vi "Receive_Log_File_FGV.vi"(7 "Session name":string, 8 "error in (no error)":errorcluster, 9 "Command":enum16{"Initialize", "Update", "Stop"}(ring), 10 "Time (ms)":u32, 11 "Processed bytes":u8[](array[numeric])) -> (0 "error out":errorcluster, 3 "Receive Log File Path":path)   [LabVIEW 2017]
uses:
  <vilib>/Utility/file.llb/Write Delimited Spreadsheet (string).vi
  <vilib>/Utility/file.llb/Write Delimited Spreadsheet (I64).vi
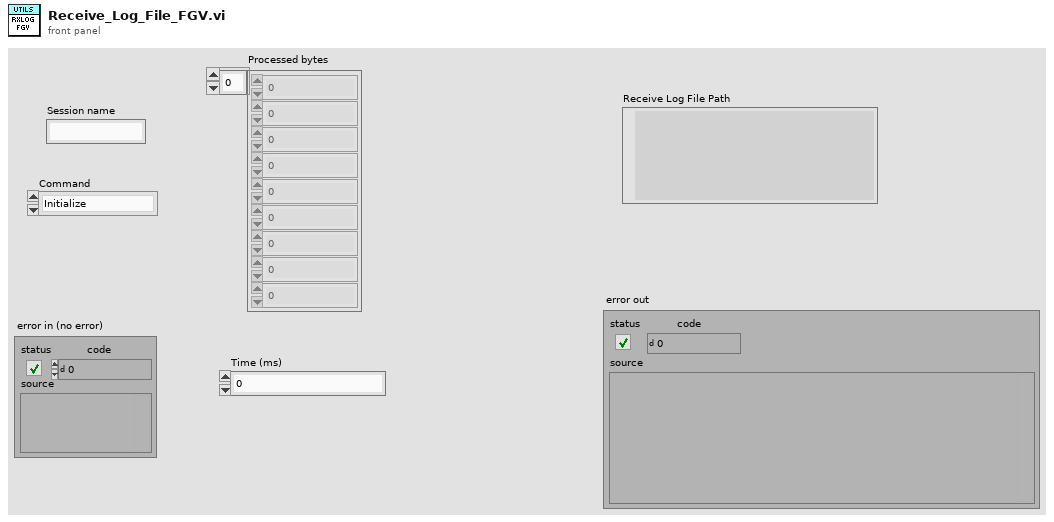
[diagram p1: front panel]
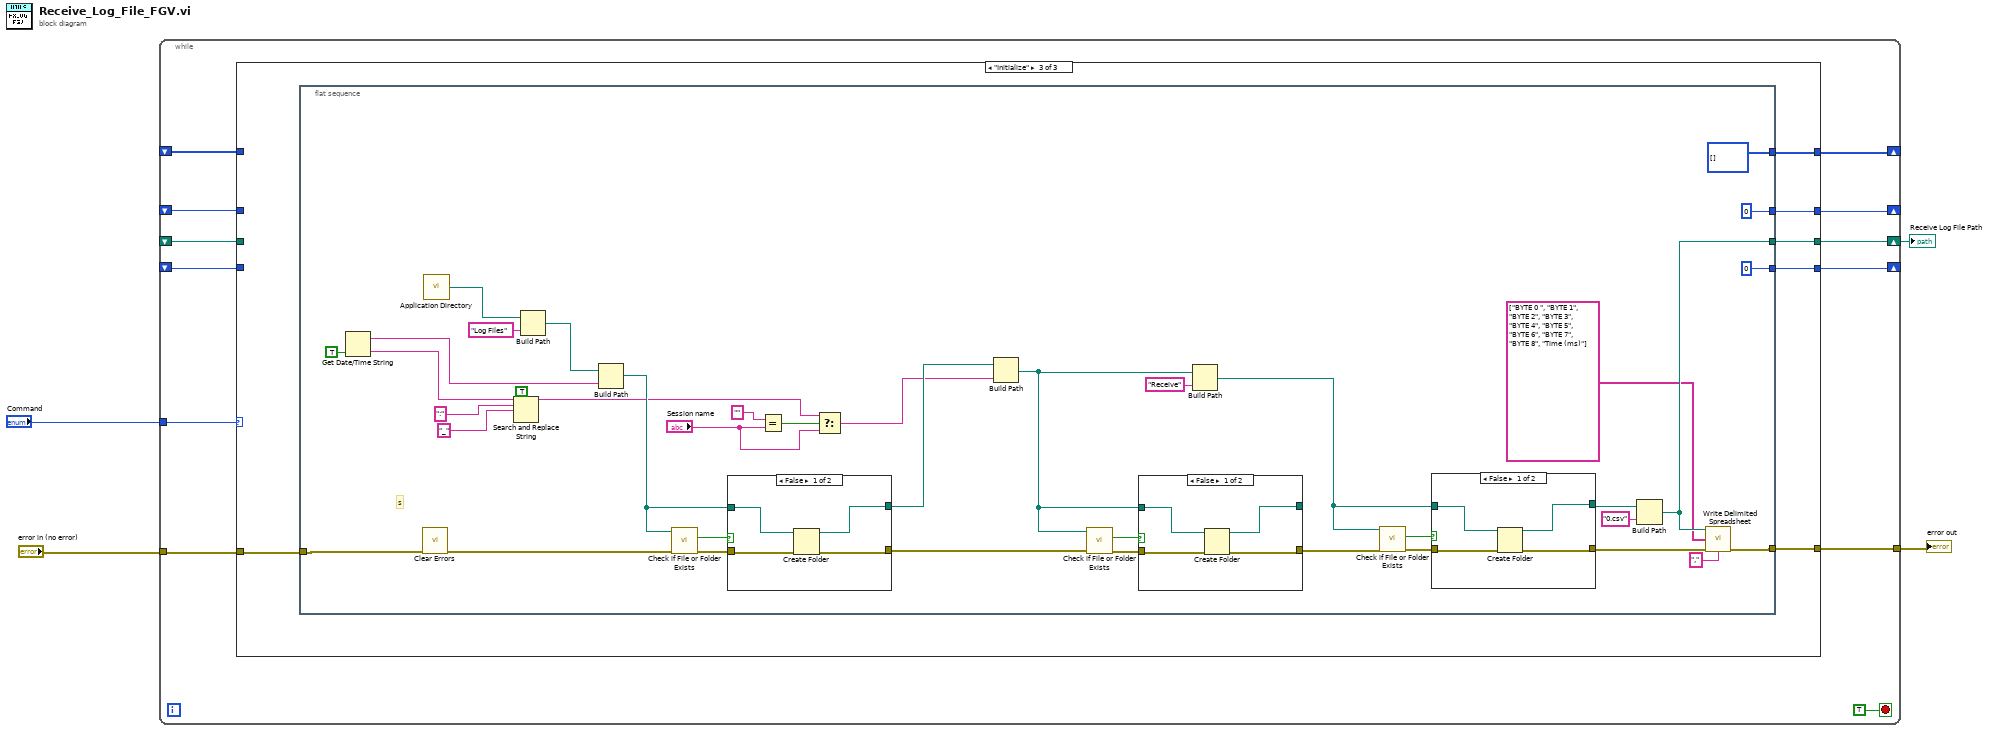
[diagram p0: block diagram]
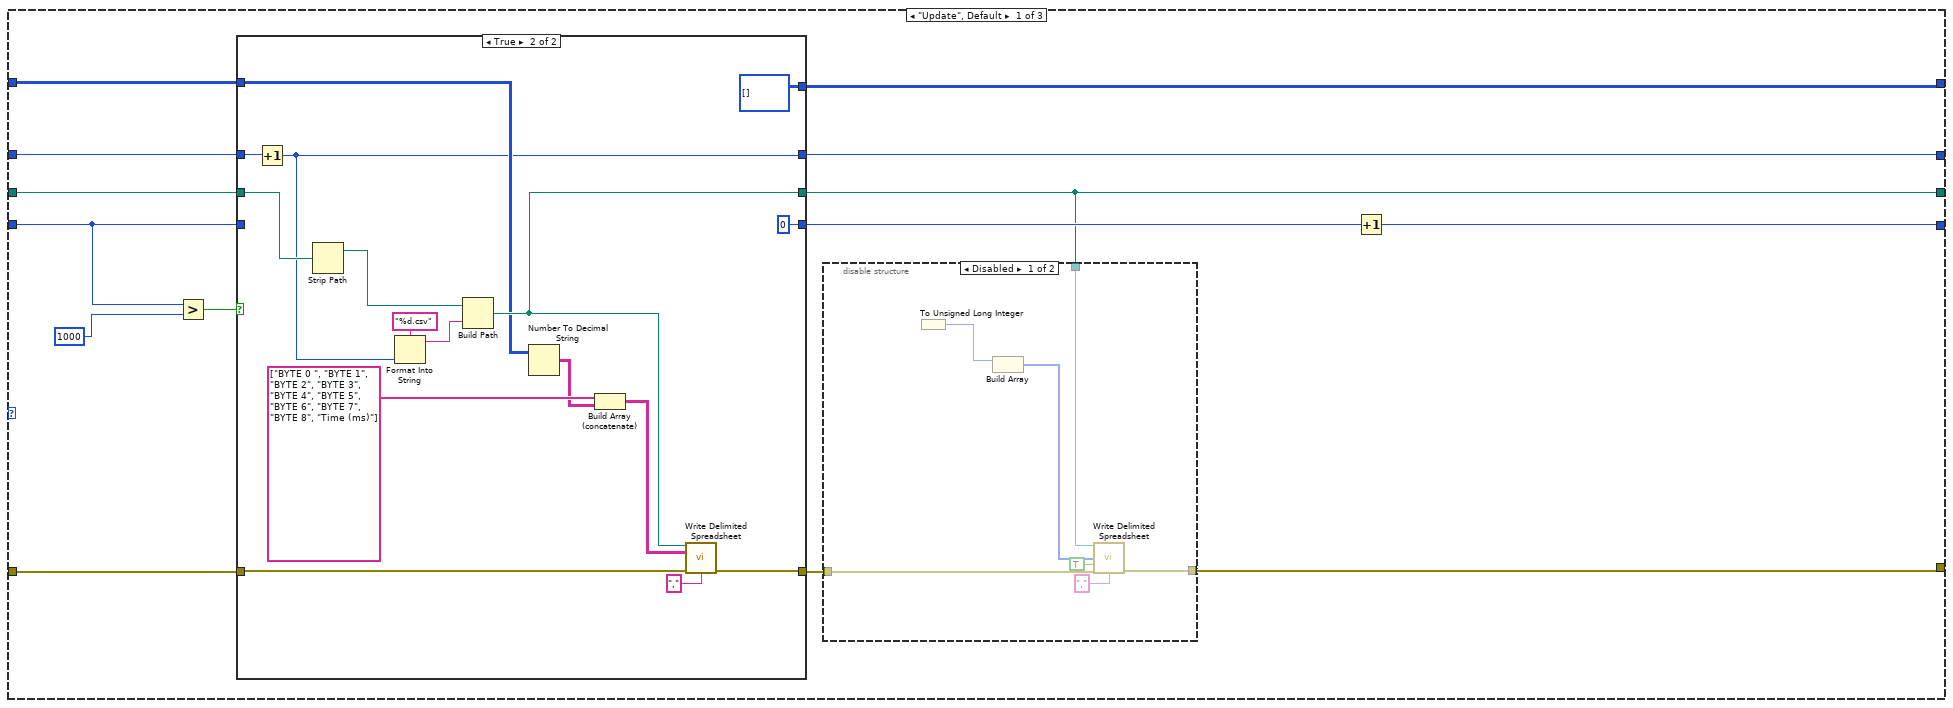
[diagram p2: hidden frame]
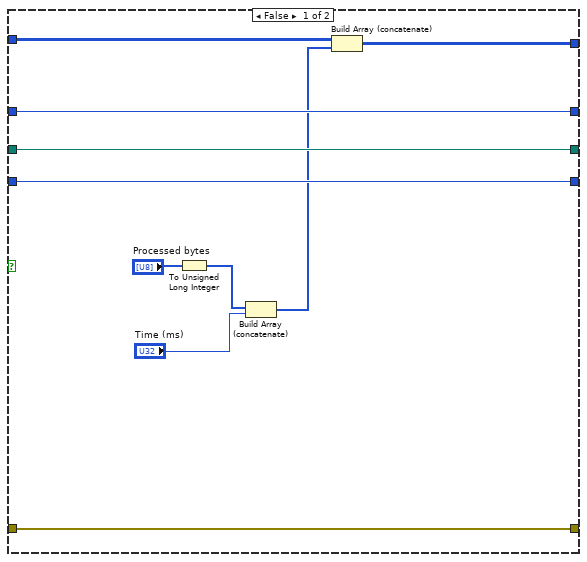
[diagram p4: hidden frame]
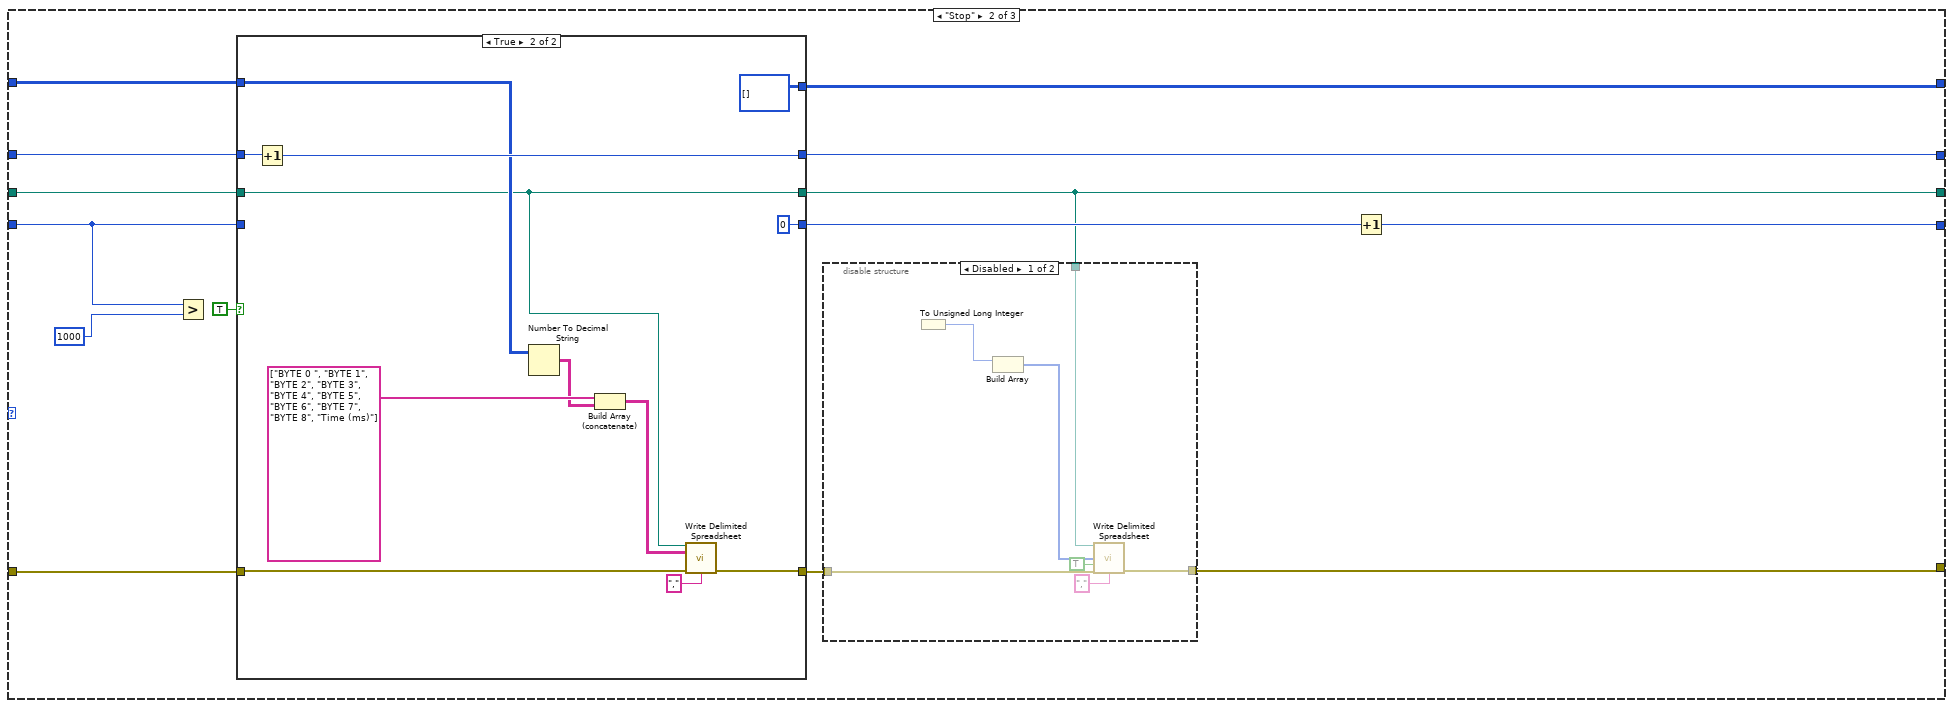
[diagram p5: hidden frame]
diagram:
  n1 = while {
    tunnel: "error in (no error)" -> [w16]
    tunnel: "Command" -> [w15]
    tunnel: [w13] -> w2
    shift-right: [w12] -> w3
    shift-left: _ -> [w9]
    shift-right: [w11] -> _
    shift-left: _ -> [w10]
    shift-right: [w8] -> _
    shift-left: _ -> [w7]
    shift-right: [w6] -> _
    shift-left: _ -> [w5]
    stop <- TRUE stop-if-true
    n2 = case shown="\"Initialize\"" w15 {
      tunnel: w16 -> [w30 w80 w113]
      tunnel: [w20 w71 w112] -> w13
      tunnel: [w21 w72 w111] -> w12
      tunnel: [w19 w70 w110] -> w11
      tunnel: w10 -> [w24 w75 _]
      tunnel: w9 -> [w27 w78 _]
      tunnel: [w25 w76 w109] -> w8
      tunnel: w7 -> [w26 w77 _]
      tunnel: [w17 w68 w108] -> w6
      tunnel: w5 -> [w18 w69 _]
      frame "Update", Default {
        n3 = Greater?(x=w24, y=1000) -> (0:w29:bool)
        n4 = case shown="True" w29 {
          tunnel: w30 -> [w49 w62]
          tunnel: [w49 w60] -> w22
          tunnel: w27 -> [w50 w66]
          tunnel: [w50 w59] -> w21
          tunnel: w26 -> [w48 w56]
          tunnel: [w48 w51] -> w25
          tunnel: w24 -> [w47 _]
          tunnel: [w47 0] -> w23
          tunnel: w18 -> [w43 w55]
          tunnel: [w41 u32[][] []] -> w17
          frame False {
            n5 = To Unsigned Long Integer(number="Processed bytes") -> (unsigned 32bit integer=w45:u32[])
            n6 = Build Array (concatenate)(w45, "Time (ms)") -> (w42:u32[])
            n7 = Build Array (concatenate)(w43, w42) -> (w41:u32[][])
          }
          frame True {
            n8 = Increment(x=w56) -> (x+1=w51:i32)
            n9 = Strip Path(path=w66) -> (stripped path=w65:path)  [unwired: 1 out]
            n10 = Format Into String(format string="%d.csv", w51) -> (resulting string=w63:string)  [unwired: 2 in, 1 out]
            n11 = Build Path(base path=w65, name or relative path=w63) -> (appended path=w59:path)
            n12 = Number To Decimal String(number=w55) -> (decimal integer string=w53:string[][])  [unwired: 1 in]
            n13 = Build Array (concatenate)(string[] ["BYTE 0 ", "BYTE 1", "BYTE 2", "BYTE 3", "BYTE 4", "BYTE 5", "BYTE 6", "BYTE 7", "BYTE 8", "Time (ms)"], w53) -> (w52:string[][])
            n14 = call-poly <vilib>:"Write Delimited Spreadsheet.vi"("file path (dialog if empty)"=w59, "2D data"=w52, "error in (no error)"=w62, "delimiter (\\t)"="," ("delimiter (\\t)")) -> ("error out"=w60:errorcluster)  [unwired: 10 in, 1 out]
          }
        }
        n15 = disable-structure shown="Disabled" {
          disable-tunnel: w22 -> [w39 w40]
          disable-tunnel: w21 -> [w38 _]
          disable-tunnel: [w35 w40] -> w20
          frame Disabled {
            n16 = To Unsigned Long Integer() -> (number=w34:u32, unsigned 32bit integer=w33:u32)
            n17 = Build Array(w33) -> (w31:u32[], w32:u32)
            n18 = call-poly <vilib>:"Write Delimited Spreadsheet.vi"("file path (dialog if empty)"=w38, "1D data"=w31, "append to file? (new file:F)"=TRUE, "error in (no error)"=w39, "delimiter (\\t)"="," ("delimiter (\\t)")) -> ("error out"=w35:errorcluster)  [unwired: 9 in, 1 out]
          }
          frame Enabled {
          }
        }
        n19 = Increment(x=w23) -> (x+1=w19:i32)
      }
      frame "Stop" {
        n20 = Greater?(x=w75, y=1000) -> ()  [unwired: 1 out]
        n21 = case shown="True" TRUE {
          tunnel: w80 -> [w94 w106]
          tunnel: [w94 w104] -> w73
          tunnel: w78 -> [w95 w96]
          tunnel: [w95 w96] -> w72
          tunnel: w77 -> [w93 w101]
          tunnel: [w93 w107] -> w76
          tunnel: w75 -> [w92 _]
          tunnel: [w92 0] -> w74
          tunnel: w69 -> [w91 w100]
          tunnel: [w91 u32[][] []] -> w68
          frame False {
          }
          frame True {
            n22 = Increment(x=w101) -> (x+1=w107:i32)
            n23 = Number To Decimal String(number=w100) -> (decimal integer string=w98:string[][])  [unwired: 1 in]
            n24 = Build Array (concatenate)(string[] ["BYTE 0 ", "BYTE 1", "BYTE 2", "BYTE 3", "BYTE 4", "BYTE 5", "BYTE 6", "BYTE 7", "BYTE 8", "Time (ms)"], w98) -> (w97:string[][])
            n25 = call-poly <vilib>:"Write Delimited Spreadsheet.vi"("file path (dialog if empty)"=w96, "2D data"=w97, "error in (no error)"=w106, "delimiter (\\t)"="," ("delimiter (\\t)")) -> ("error out"=w104:errorcluster)  [unwired: 10 in, 1 out]
          }
        }
        n26 = disable-structure shown="Disabled" {
          disable-tunnel: w73 -> [w89 w90]
          disable-tunnel: w72 -> [w88 _]
          disable-tunnel: [w85 w90] -> w71
          frame Disabled {
            n27 = To Unsigned Long Integer() -> (number=w84:u32, unsigned 32bit integer=w83:u32)
            n28 = Build Array(w83) -> (w81:u32[], w82:u32)
            n29 = call-poly <vilib>:"Write Delimited Spreadsheet.vi"("file path (dialog if empty)"=w88, "1D data"=w81, "append to file? (new file:F)"=TRUE, "error in (no error)"=w89, "delimiter (\\t)"="," ("delimiter (\\t)")) -> ("error out"=w85:errorcluster)  [unwired: 9 in, 1 out]
          }
          frame Enabled {
          }
        }
        n30 = Increment(x=w74) -> (x+1=w70:i32)
      }
      frame "Initialize" {
        n31 = flat-sequence {
          tunnel: w113 -> [w115]
          tunnel: [w125] -> w112
          tunnel: [w127] -> w111
          tunnel: [0] -> w110
          tunnel: [0] -> w109
          tunnel: [u32[][] []] -> w108
          frame #0 {
            # "s"
            n32 = Get Date/Time String(want seconds? (F)=TRUE) -> (date string=w148:string, time string=w143:string)  [unwired: 2 in]
            n33 = call <vilib>:"Clear Errors.vi"("error in (no error)"=w115) -> ("error out"=w114:errorcluster)  [unwired: 5 in, 1 out]
            n34 = call <vilib>:"Application Directory.vi"() -> ("Application Directory"=w151:path)
            n35 = Search and Replace String(replace all?=TRUE ("replace all? (F)"), input string=w143, search string=":", replace string="_" ("replace string (\"\")")) -> (result string=w119:string)  [unwired: 4 in, 3 out]
            n36 = Build Path(base path=w151, name or relative path="Log Files") -> (appended path=w149:path)
            n37 = Build Path(base path=w149, name or relative path=w148) -> (appended path=w145:path)
            n38 = call <vilib>:"Check if File or Folder Exists.vi"("error in (no error)"=w114, "path"=w145) -> ("error out"=w146:errorcluster, "file or folder exists?"=w147:bool)  [unwired: 7 in, 1 out]
            n39 = case shown="False" w147 {
              tunnel: w146 -> [w168 w170]
              tunnel: [w166 w170] -> w137
              tunnel: w145 -> [w167 w169]
              tunnel: [w165 w169] -> w144
              frame False {
                n40 = Create Folder(path (use dialog)=w167, error in=w168) -> (created path=w165:path, error out=w166:errorcluster)  [unwired: 1 in, 1 out]
              }
              frame True {
              }
            }
            n41 = Equal?(x="", y="Session name") -> (x = y?=w120:bool)
            n42 = Select(t=w119, s=w120, f="Session name") -> (s? t:f=w118:string)
            n43 = Build Path(base path=w144, name or relative path=w118) -> (appended path=w136:path)
            n44 = call <vilib>:"Check if File or Folder Exists.vi"("error in (no error)"=w137, "path"=w136) -> ("error out"=w138:errorcluster, "file or folder exists?"=w139:bool)  [unwired: 7 in, 1 out]
            n45 = case shown="False" w139 {
              tunnel: w138 -> [w162 w164]
              tunnel: [w160 w164] -> w132
              tunnel: w136 -> [w161 w163]
              tunnel: [w159 w163] -> _
              frame False {
                n46 = Create Folder(path (use dialog)=w161, error in=w162) -> (created path=w159:path, error out=w160:errorcluster)  [unwired: 1 in, 1 out]
              }
              frame True {
              }
            }
            n47 = Build Path(base path=w136, name or relative path="Receive") -> (appended path=w131:path)
            n48 = call <vilib>:"Check if File or Folder Exists.vi"("error in (no error)"=w132, "path"=w131) -> ("error out"=w133:errorcluster, "file or folder exists?"=w134:bool)  [unwired: 7 in, 1 out]
            n49 = case shown="False" w134 {
              tunnel: w133 -> [w156 w158]
              tunnel: [w154 w158] -> w130
              tunnel: w131 -> [w155 w157]
              tunnel: [w153 w157] -> w129
              frame False {
                n50 = Create Folder(path (use dialog)=w155, error in=w156) -> (created path=w153:path, error out=w154:errorcluster)  [unwired: 1 in, 1 out]
              }
              frame True {
              }
            }
            n51 = Build Path(base path=w129, name or relative path="0.csv") -> (appended path=w127:path)
            n52 = call-poly <vilib>:"Write Delimited Spreadsheet.vi"("file path (dialog if empty)"=w127, "1D data"=string[] ["BYTE 0 ", "BYTE 1", "BYTE 2", "BYTE 3", "BYTE 4", "BYTE 5", "BYTE 6", "BYTE 7", "BYTE 8", "Time (ms)"], "error in (no error)"=w130, "delimiter (\\t)"="," ("delimiter (\\t)")) -> ("error out"=w125:errorcluster)  [unwired: 10 in, 1 out]
          }
        }
      }
    }
  }
  "error out" <- w2
  "Receive Log File Path" <- w3
